vi "Configure Trigger.vi"(5 "Trigger Mode (0:Auto)":i32(ring) items=["Auto", "Normal", "OFF"], 7 "Synchronization Source (0: U1)":i32(ring) items=["U1", "I1", "U2", "I2", "U3", "I3", "U4", "I4", "U5", "I5", "U6", "I6", "External Clock"], 8 "error in (no error)":errorcluster, 9 "Trigger Level (0.0 %)":dbl min=-100.0 max=100.0 format="%.1f", 10 "Trigger Slope (0: Rise)":i32(ring) items=["Rise", "Fall", "Both"], 11 "VISA resource name":refnum<visa-resource-name>) -> (0 "error out":errorcluster, 3 "VISA resource name out":refnum<visa-resource-name>)   [LabVIEW 2021, in "Yokogawa WT1800 Series.lvlib"]
doc: "Configures the trigger features."
uses:
  <instrlib>/Yokogawa WT1800 Series/Yokogawa WT1800 Series.lvlib
panel:
  # "%"
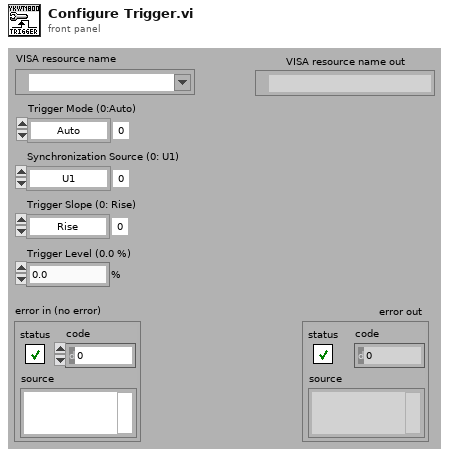
[diagram p1: front panel]
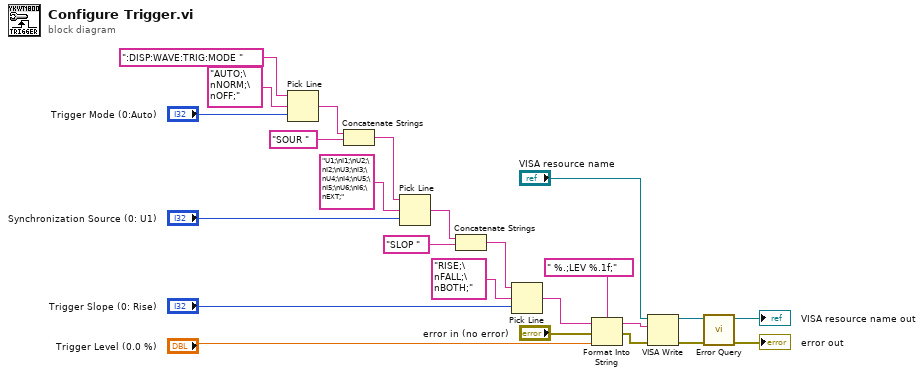
[diagram p0: block diagram]
diagram:
  n1 = Pick Line ("ライン選択")(string ("")=":DISP:WAVE:TRIG:MODE " ("¶ñi\"\"j"), multi-line string="AUTO;\nNORM;\nOFF;" ("複数行文字列"), line index="Trigger Mode (0:Auto)") -> (output string=w13:string)
  n2 = Concatenate Strings(w13, "SOUR " ("形式文字列")) -> (w12:string)
  n3 = Pick Line ("ライン選択")(string ("")=w12, multi-line string="U1;\nI1;\nU2;\nI2;\nU3;\nI3;\nU4;\nI4;\nU5;\nI5;\nU6;\nI6;\nEXT;" ("複数行文字列"), line index="Synchronization Source (0: U1)") -> (output string=w8:string)
  n4 = Concatenate Strings(w8, "SLOP " ("形式文字列")) -> (w7:string)
  n5 = Pick Line ("ライン選択")(string ("")=w7, multi-line string="RISE;\nFALL;\nBOTH;" ("複数行文字列"), line index="Trigger Slope (0: Rise)") -> (output string=w4:string)
  n6 = Format Into String(format string=" %.;LEV %.1f;" ("形式文字列"), initial string=w4, error in="error in (no error)", "Trigger Level (0.0 %)") -> (resulting string=w2:string, error out=w1:errorcluster)
  n7 = VISA Write ("VISA書き込み")(VISA resource name="VISA resource name", write buffer=w2, error in (no error)=w1) -> (VISA resource name out=w24:refnum<visa-resource-name>, error out=w23:errorcluster)  [unwired: 1 out]
  n8 = call <instrlib>:"Error Query.vi"("error in (no error)"=w23, "VISA resource name"=w24) -> ("error out"=→"error out":errorcluster, "VISA resource name out"=→"VISA resource name out":refnum<visa-resource-name>)  [unwired: 6 in, 2 out]
